vi "test Should Return Multiple Call Parameters In The Same Order As Called.vi"(8 "error in (no error)":errorcluster, 11 "TestCase in":refnum<class "Store and Return Parameters.lvclass">) -> (0 "error out":errorcluster, 3 "TestCase out":refnum<class "Store and Return Parameters.lvclass">)   [LabVIEW 2013, in "Store and Return Parameters.lvclass"]
uses:
  Store and Return Parameters.lvclass
  Core Classes/LabSpy/LabSpy.lvclass
  <vilib>/addons/_JKI Toolkits/VI Tester/TestCase.llb/TestCase.lvclass
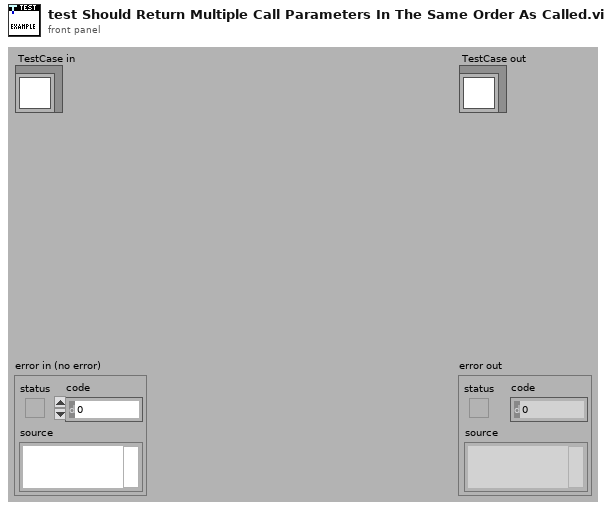
[diagram p1: front panel]
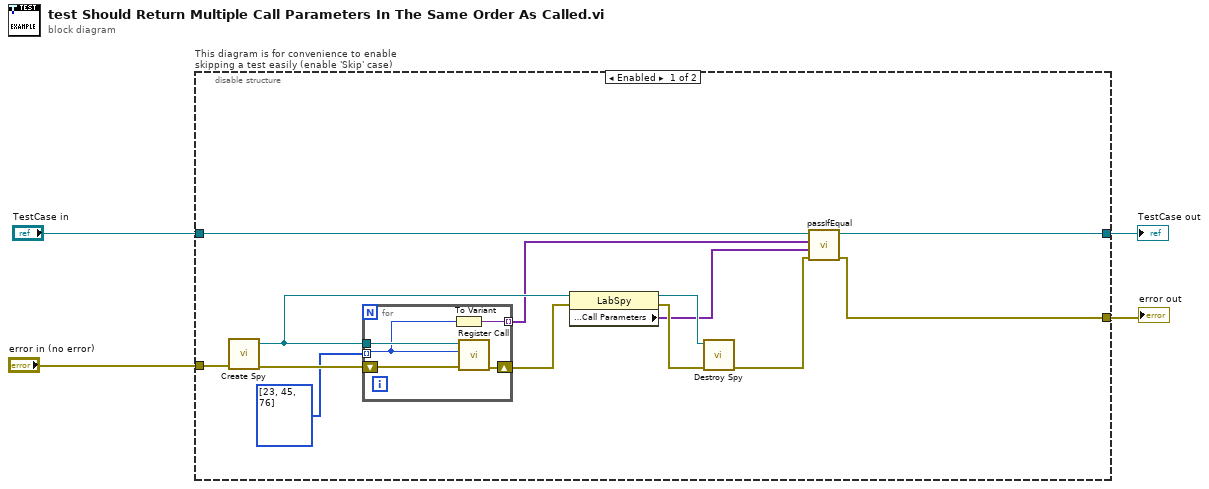
[diagram p0: block diagram]
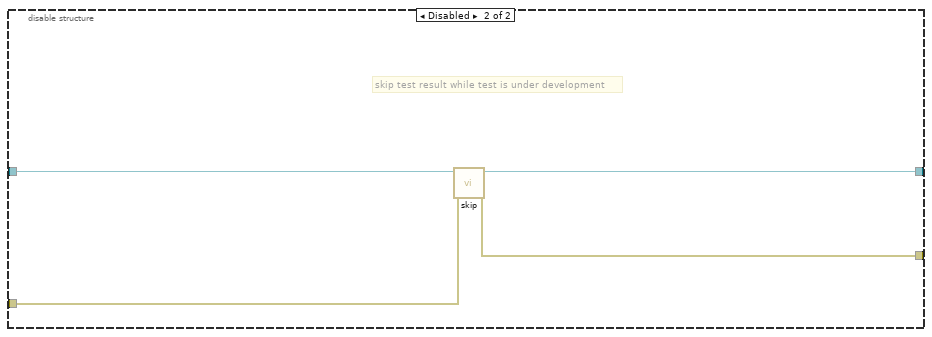
[diagram p2: hidden frame]
diagram:
  n1 = disable-structure "This diagram is for convenience to enable skipping a test easily (enable 'Skip' case)" shown="Enabled" {
    disable-tunnel: "TestCase in" -> [w11 w26]
    disable-tunnel: [w10 w24] -> w1
    disable-tunnel: [w9 w25] -> w3
    disable-tunnel: "error in (no error)" -> [w17 w23]
    frame Enabled {
      n2 = call "Create Spy.vi"("error in (no error)"=w17) -> ("error out"=w16:errorcluster, "LabSpy Out"=w15:refnum<data-value>)  [unwired: 9 in]
      n3 = for {
        tunnel: w15 -> [w21]
        shift-right: [w20] -> w14
        shift-left: w16 -> [w22]
        tunnel: i32[] [23, 45, 76] -> [w19] mode=indexing
        tunnel: [w18] -> w5 mode=indexing
        n4 = To Variant(anything=w19) -> (Variant=w18:variant)
        n5 = call "Register Call.vi"("error in (no error)"=w22, "Parameters"=w19, "LabSpy"=w21) -> ("error out"=w20:errorcluster)  [unwired: 7 in, 1 out]
      }
      n6 = property class="LabSpy"(reference=w15, error in=w14) -> (reference out=w12:refnum<data-value>, error out=w13:errorcluster, "Parameter Readings:Call Parameters"=w7:variant[])
      n7 = call "Destroy Spy.vi"("error in (no error)"=w13, "LabSpy"=w12) -> ("error out"=w8:errorcluster)  [unwired: 9 in]
      n8 = call-dynamic "passIfEqual.vi"("error in (no error)"=w8, "y"=w7, "x"=w5, "TestCase in"=w11) -> ("error out"=w9:errorcluster, "TestCase out"=w10:refnum<class "Store and Return Parameters.lvclass">)  [unwired: 6 in]
    }
    frame Disabled {
      # "skip test result while test is under development"
      n9 = call <vilib>:"skip.vi"("error in (no error)"=w23, "TestCase in"=w26) -> ("error out"=w25:errorcluster, "TestCase out"=w24:refnum<class "Store and Return Parameters.lvclass">)  [unwired: 8 in]
    }
  }
  "error out" <- w3
  "TestCase out" <- w1
